vi "CalculateTeperature.vi"(8 "error in (no error)":errorcluster, 10 "Resistor":dbl, 11 "ChannelVoltage":dbl) -> (0 "error out":errorcluster, 3 "Temperature":dbl)   [LabVIEW 2017]
uses:
  <vilib>/express/express arith-compare/Formula/XNode/ExpressFormulaBlockNode.xnode
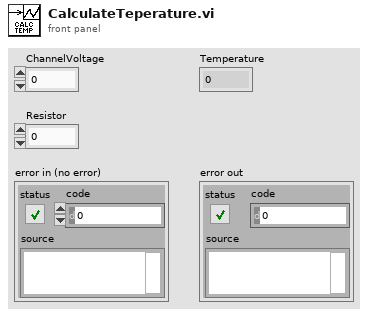
[diagram p1: front panel]
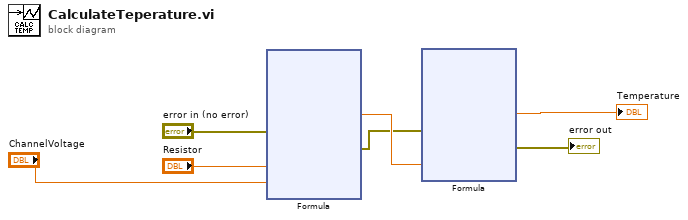
[diagram p0: block diagram]
diagram:
  n1 = xnode "Formula"("error in (no error)"="error in (no error)", "Rresistor"="Resistor", "Vtherm"="ChannelVoltage") -> ("Result"=w5:dbl, "error out"=w4:errorcluster)
  n2 = xnode "Formula"("error in (no error)"=w4, "Rresistor"=w5) -> ("Result"=→"Temperature":dbl, "error out"=→"error out":errorcluster)
